vi "Read Data.vi"(8 "error in (no error)":errorcluster caption="错误输入（无错误）", 11 "DAM0200-Relay 输入":refnum<class "DAM0200-Relay.lvclass">) -> (0 "error out":errorcluster caption="错误输出", 3 "DAM0200-Relay 输出":refnum<class "DAM0200-Relay.lvclass">)   [LabVIEW 2016, in "DAM0200-Relay.lvlib" / "DAM0200-Relay.lvclass"]
uses:
  DAM0200-Relay.lvclass
  DAM0200-Relay.lvclass/DAM0200-Relay.ctl
  <vilib>/Plasmionique/MB Master/MB Master.lvlib
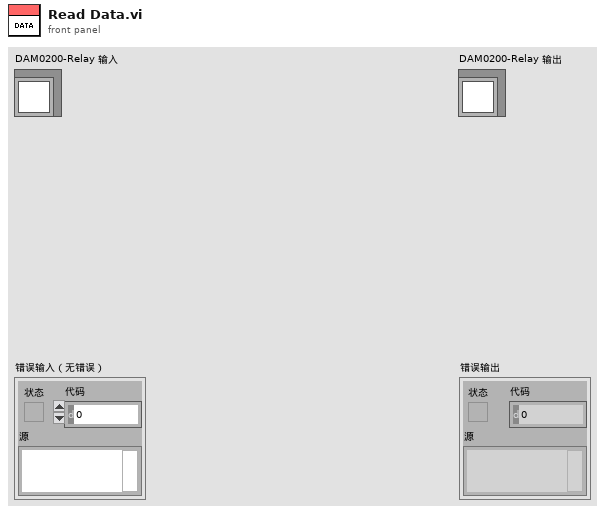
[diagram p1: front panel]
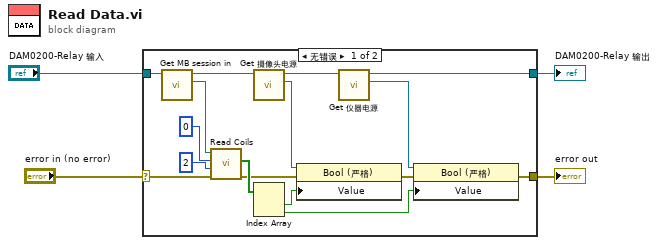
[diagram p0: block diagram]
diagram:
  n1 = case shown="无错误" "error in (no error)" {
    selector: "error in (no error)" -> [w16 w22]
    tunnel: [w5 w22] -> w3
    tunnel: [w7 w21] -> w1
    tunnel: "DAM0200-Relay 输入" -> [w20 w21]
    frame No Error {
      n2 = call "Get MB session in.vi"("DAM0200-Relay in"=w20) -> ("MB Serial Master:MB_Master"=w17:refnum<class "MB_Master.lvclass">, "DAM0200-Relay out"=w19:refnum<class "DAM0200-Relay.lvclass">)  [unwired: 9 in]
      n3 = call <vilib>:"Read Coils.vi"("error in (no error)"=w16, "quantity"=u16 2, "starting address"=u16 0, "MB session in"=w17) -> ("error out"=w6:errorcluster, "Coils"=w13:bool[])  [unwired: 5 in, 1 out]
      n4 = call "Get 摄像头电源.vi"("DAM0200-Relay in"=w19) -> ("摄像头电源"=w12:refnum<vi>, "DAM0200-Relay out"=w18:refnum<class "DAM0200-Relay.lvclass">)  [unwired: 9 in]
      n5 = Index Array(array=w13) -> (element #1=w11:bool, element #2=w8:bool)  [unwired: 2 in]
      n6 = property class="Bool (严格)"(reference=w12, error in=w6, "Value"=w11) -> (error out=w10:errorcluster)  [unwired: 1 out]
      n7 = call "Get 仪器电源.vi"("DAM0200-Relay in"=w18) -> ("仪器电源"=w9:refnum<vi>, "DAM0200-Relay out"=w7:refnum<class "DAM0200-Relay.lvclass">)  [unwired: 9 in]
      n8 = property class="Bool (严格)"(reference=w9, error in=w10, "Value"=w8) -> (error out=w5:errorcluster)  [unwired: 1 out]
    }
    frame Error {
    }
  }
  "error out" <- w3
  "DAM0200-Relay 输出" <- w1
